vi "GraphsUpdateProc.vi"(10 "Compiler Settings":T1={"Python Path"=path "", "Main File"="mainscript.py", "Meta File"="metascript.txt", "Aux File"="auxscript.py", "Pre File"="metascript.txt"}, 11 "proc graph ref":refnum<vi>) -> (2 "SaveToCSV?":bool=TRUE, 3 "Array":dbl[][](array[numeric]))   [LabVIEW 2019]
uses:
  PulseCompiler/CompilerSettings.ctl
  controls/GlobalExp.vi
  Global.lvlib
panel:
  in  "error in (no error)":errorcluster
  out "error out":errorcluster
  out "value 2":string
  out "return code":i32
  out "standard error":string
  out "standard output":string
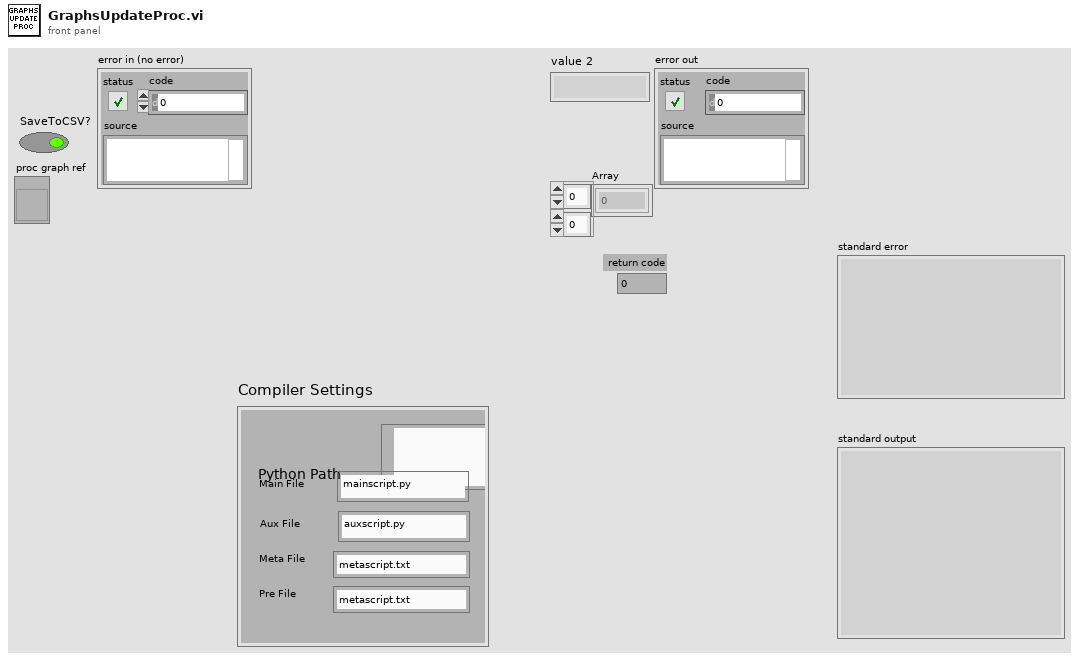
[diagram p1: front panel]
types:
  T1 = typedef "CompilerSettings.ctl" = cluster{"Python Path":path, "Main File":string, "Meta File":string, "Aux File":string, "Pre File":string}
  T2 = typedef "MasterExpControl.ctl" = cluster{"Main Steps":dbl, "Main Runs":dbl, "ExpStatus":enum16{"Innit", "Stop", "Idle", "MainRunning", "AuxRunning"}, "Main Current Step":dbl, "ExpNum":dbl, "NewData":bool, "date":string, "command":string, "Stop":bool, "Pause":bool, "Mathematica":string, "Main/Meta":bool, "UpdateMath":bool, "Camera":bool, "MetaExpOver":bool, "NextMetaExp":bool}
  T3 = cluster{"date":string, "expnum":string, "save":i32}
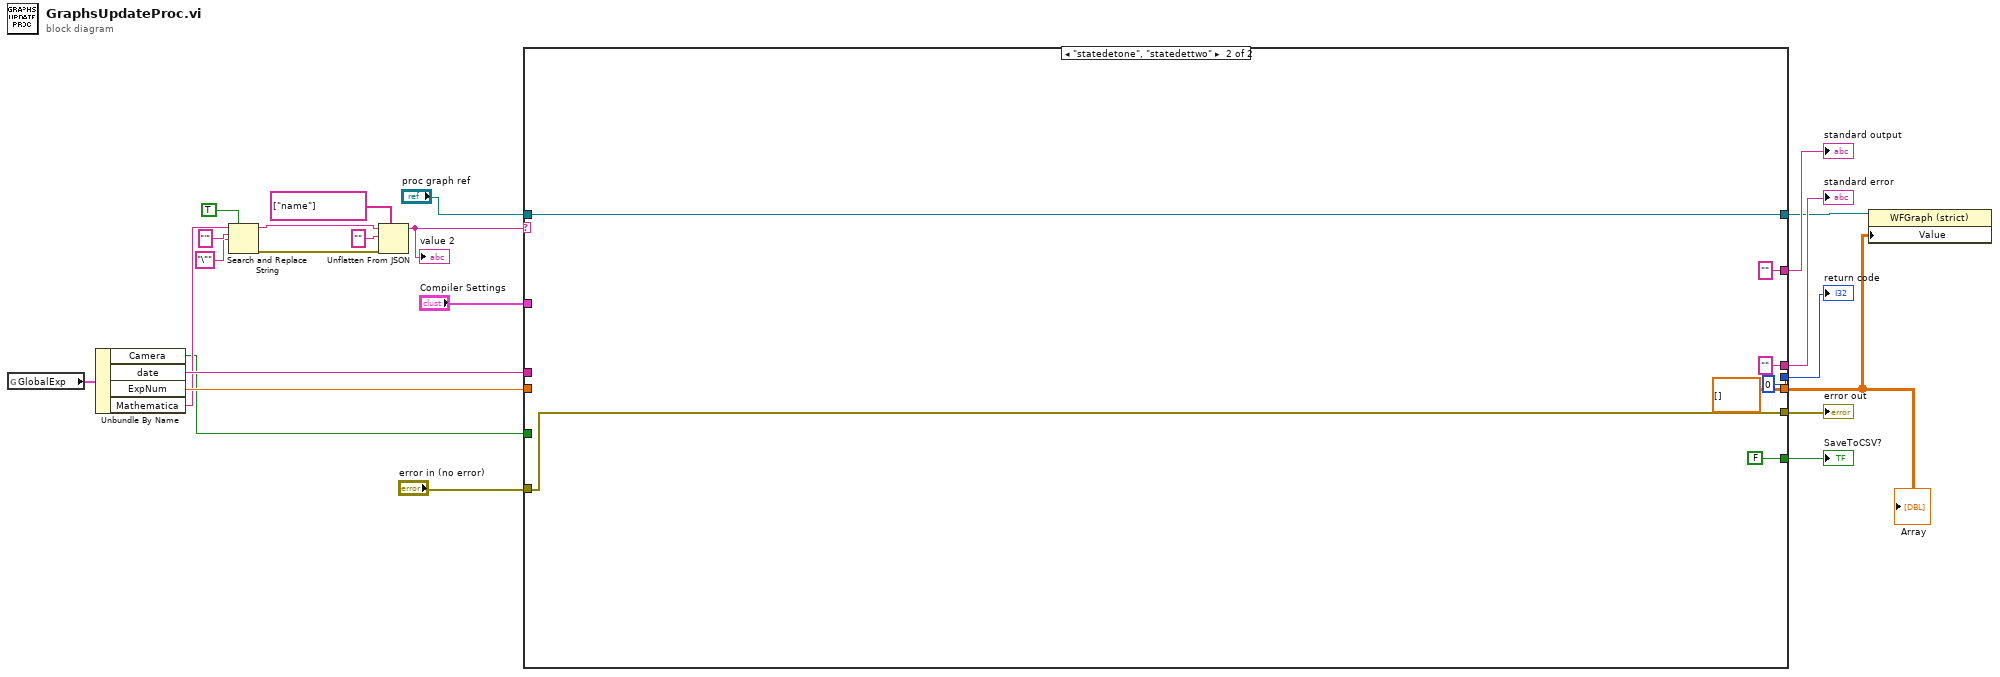
[diagram p0: block diagram]
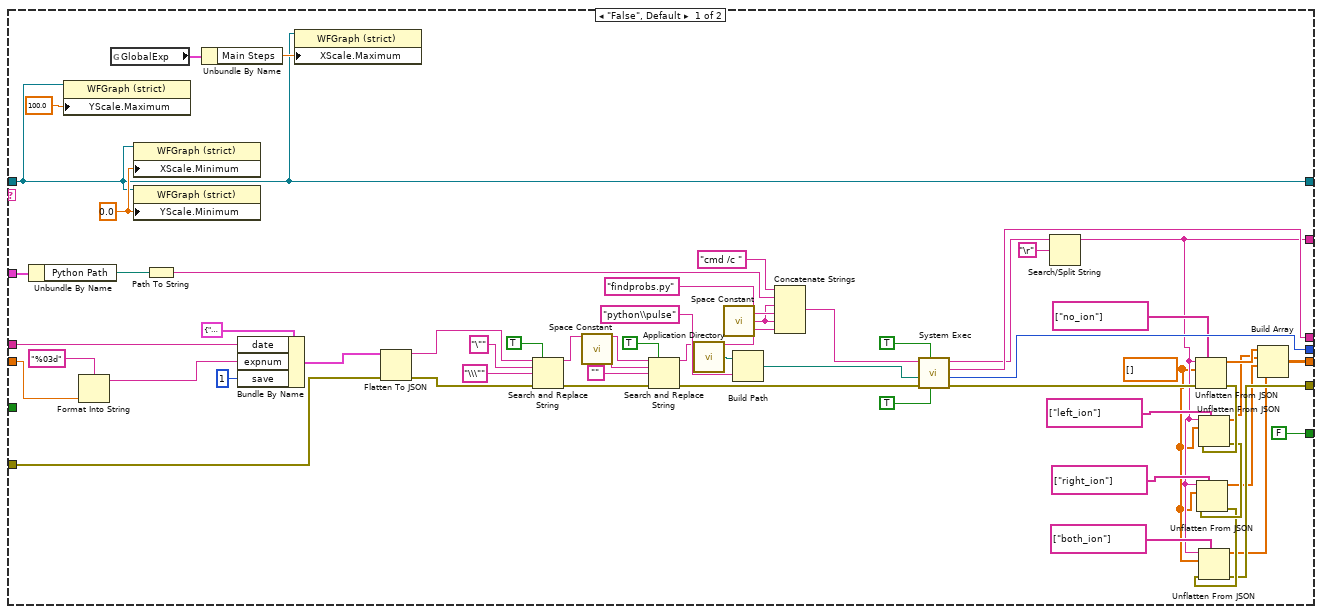
[diagram p2: hidden frame]
diagram:
  n1 = global read "GlobalExp.vi" "GlobalExp"() -> (w20:T2)
  n2 = Unbundle By Name(w20) -> ("Camera"=w6:bool, "date"=w19:string, "ExpNum"=w18:dbl, "Mathematica"=w12:string)
  n3 = Search and Replace String(replace all?=TRUE ("replace all? (F)"), input string=w12, search string="'", replace string="\"" ("replace string (\"\")")) -> (result string=w8:string, error out=w9:errorcluster)  [unwired: 4 in, 2 out]
  n4 = Unflatten From JSON(path=string[] ["name"], JSON string=w8, type and defaults="", error in (no error)=w9) -> (value=w7:string)  [unwired: 3 in, 1 out]
  "value 2" <- w7
  n5 = case shown="\"statedetone\", \"statedettwo\"" w7 {
    tunnel: [w81 "" ("standard error")] -> w23
    tunnel: [w70 0 ("return code")] -> w22
    tunnel: [w34 "" ("standard output")] -> w21
    tunnel: [w24 dbl[][] []] -> w2
    tunnel: w19 -> [w53 _]
    tunnel: w18 -> [w51 _]
    tunnel: [w42 w87] -> w17
    tunnel: "proc graph ref" -> [w42 w87]
    tunnel: [FALSE FALSE] -> w16
    tunnel: [w29 w83] -> w5
    tunnel: w6 -> [_ _]
    tunnel: "Compiler Settings" -> [w40 _]
    tunnel: "error in (no error)" -> [w38 w83]
    frame "False", Default {
      w46 = 0.0 ("X Scale.Range:Minimum")
      w33 = dbl[] []
      n6 = Unbundle By Name(w40) -> ("Python Path"=w44:path)
      n7 = property class="WFGraph (strict)"(reference=w42, "YScale.Maximum"=100.0 ("Y Scale.Range:Maximum")) -> ()  [unwired: 1 in, 2 out]
      n8 = Format Into String(format string="%03d", w51) -> (resulting string=w52:string)  [unwired: 2 in, 1 out]
      n9 = global read "GlobalExp.vi" "GlobalExp"() -> (w48:T2)
      n10 = property class="WFGraph (strict)"(reference=w42, "XScale.Minimum"=w46) -> ()  [unwired: 1 in, 2 out]
      n11 = property class="WFGraph (strict)"(reference=w42, "YScale.Minimum"=w46) -> ()  [unwired: 1 in, 2 out]
      n12 = Path To String(path=w44) -> (string=w43:string)
      n13 = Unbundle By Name(w48) -> ("Main Steps"=w47:dbl)
      n14 = Bundle By Name(cluster=T3 {"date"="", "expnum"="", "save"=0}, "date"=w53, "expnum"=w52, "save"=1) -> (w54:T3)
      n15 = property class="WFGraph (strict)"(reference=w42, "XScale.Maximum"=w47) -> ()  [unwired: 1 in, 2 out]
      n16 = Flatten To JSON(anything=w54, error in (no error)=w38) -> (JSON string=w67:string, 11:w66:errorcluster)  [unwired: 1 in]
      n17 = Search and Replace String(replace all?=TRUE ("replace all? (F)"), input string=w67, search string="\"", replace string="\\\"" ("replace string (\"\")"), error in=w66) -> (result string=w63:string, error out=w62:errorcluster)  [unwired: 3 in, 2 out]
      n18 = call <vilib>:"Space Constant.vi"() -> ("String"=w61:string)
      n19 = Search and Replace String(replace all?=TRUE ("replace all? (F)"), input string=w63, search string=w61, replace string="", error in=w62) -> (result string=w59:string, error out=w58:errorcluster)  [unwired: 3 in, 2 out]
      n20 = call <vilib>:"Application Directory.vi"() -> ("Application Directory"=w75:path)
      n21 = call <vilib>:"Space Constant.vi"() -> ("String"=w68:string)
      n22 = Build Path(base path=w75, name or relative path="python\\pulse") -> (appended path=w77:path)
      n23 = Concatenate Strings("cmd /c " ("string"), w43, w68, "findprobs.py" ("name or relative path"), w68, w59) -> (w72:string)
      n24 = call <vilib>:"System Exec.vi"("run minimized? (F)"=TRUE, "wait until completion? (T)"=TRUE, "error in (no error)"=w58, "working directory"=w77, "command line"=w72) -> ("error out"=w49:errorcluster, "return code"=w70:i32, "standard error"=w81:string, "standard output"=w73:string)  [unwired: 3 in]
      n25 = Search/Split String(string=w73, search string/char (-)="\r") -> (substring before match=w34:string)  [unwired: 1 in, 2 out]
      n26 = Unflatten From JSON(path=string[] ["no_ion"], JSON string=w34, type and defaults=w33, error in (no error)=w49) -> (value=w28:dbl[], error out=w32:errorcluster)  [unwired: 3 in]
      n27 = Unflatten From JSON(path=string[] ["left_ion"], JSON string=w34, type and defaults=w33, error in (no error)=w32) -> (value=w27:dbl[], error out=w31:errorcluster)  [unwired: 3 in]
      n28 = Unflatten From JSON(path=string[] ["right_ion"], JSON string=w34, type and defaults=w33, error in (no error)=w31) -> (value=w26:dbl[], error out=w30:errorcluster)  [unwired: 3 in]
      n29 = Unflatten From JSON(path=string[] ["both_ion"], JSON string=w34, type and defaults=w33, error in (no error)=w30) -> (value=w25:dbl[], error out=w29:errorcluster)  [unwired: 3 in]
      n30 = Build Array(w28, w27, w26, w25) -> (w24:dbl[][])
    }
    frame "statedetone", "statedettwo" {
    }
  }
  "standard output" <- w21
  "standard error" <- w23
  "return code" <- w22
  "SaveToCSV?" <- w16
  "error out" <- w5
  "Array" <- w2
  n31 = property class="WFGraph (strict)"(reference=w17, "Value"=w2) -> ()  [unwired: 1 in, 2 out]
